vi "Activate Remote Trace.vi"(8 "error in (no error)":errorcluster, 10 "Remote Trace (On)":bool=TRUE, 11 "VISA resource name":refnum<visa-resource-name>) -> (0 "error out":errorcluster, 3 "VISA resource name out":refnum<visa-resource-name>)   [LabVIEW 2020, in "Rohde&Schwarz CMXP Base.lvlib"]
doc: "Enables tracing.\n\nAttribute:\nRSCMXPBASE_ATTR_REMOTE_TRACE_ACTIVE\n\nRemote-control command:\n[CONFigure:]BASE:RTRace:ACTive"
uses:
  <instrlib>/Rohde&Schwarz CMXP Base/Rohde&Schwarz CMXP Base.lvlib
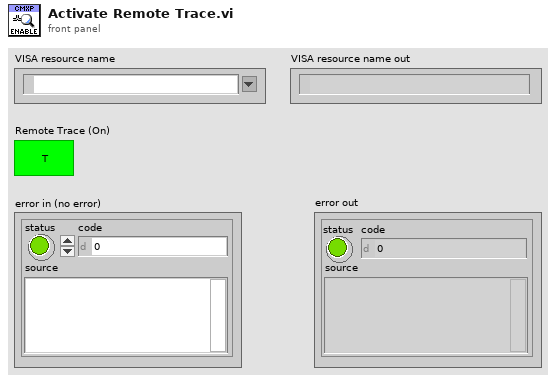
[diagram p1: front panel]
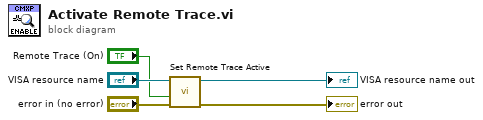
[diagram p0: block diagram]
diagram:
  n1 = call "Set Remote Trace Active"("error in (no error)"="error in (no error)", "Remote Trace Active (OFF)"="Remote Trace (On)", "instrument handle"="VISA resource name") -> ("error out"=→"error out":errorcluster, "instrument handle out"=→"VISA resource name out":refnum<visa-resource-name>)  [unwired: 7 in]
